vi "MccHat_extract_pressure_SPT25.vi"(8 "readings":cluster{i32, i32, dbl}[](array[cluster]), 11 "time":timestamp) -> (2 "P":dbl, 3 "waveform_array":waveform(dbl)[](array[waveform])=[{"t0"=timestamp(0 s since 1904-01-01), "dt"=1.0, "Y"=[]}, {"t0"=timestamp(3732035173.078092 s since 1904-01-01), "dt"=1.0, "Y"=[302.8589782714844], "attributes"=variant("NI_ChannelName"=variant(string "T1"))}])   [LabVIEW 2019]
panel:
  in  "V_max":dbl=10.0
  in  "V_min":dbl
  in  "P_max":dbl=30.0
  in  "P_min":dbl=-14.7
  out "V":dbl
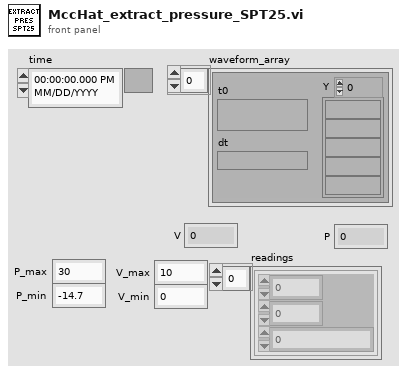
[diagram p1: front panel]
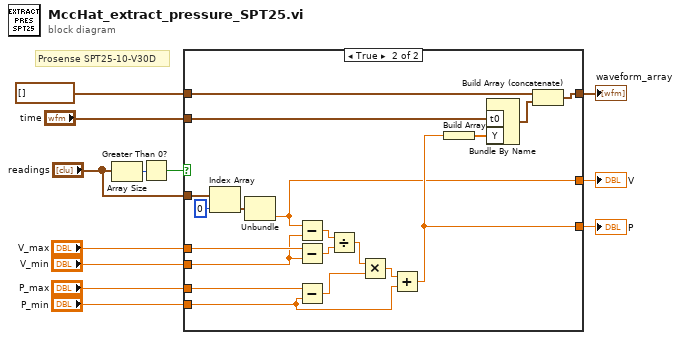
[diagram p0: block diagram]
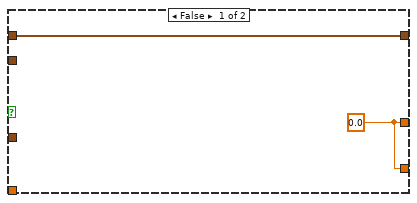
[diagram p2: hidden frame]
diagram:
  # "Prosense SPT25-10-V30D"
  n1 = Array Size(array="readings") -> (size(s)=w2:i32)
  n2 = Greater Than 0?(x=w2) -> (x > 0?=w12:bool)
  n3 = case shown="True" w12 {
    tunnel: waveform(dbl)[] [] -> [w14 w33]
    tunnel: "time" -> [_ w32]
    tunnel: [w14 w31] -> w9
    tunnel: [w13 w19] -> w8
    tunnel: [w13 w15] -> w7
    tunnel: "P_min" -> [_ w20]
    tunnel: "P_max" -> [_ w24]
    tunnel: "V_max" -> [_ w28]
    tunnel: "V_min" -> [_ w27]
    tunnel: "readings" -> [_ w18]
    frame False {
      w13 = 0.0 ("CJC (K)")
    }
    frame True {
      n4 = Index Array(array=w18, index=0) -> (element=w16:cluster{i32, i32, dbl})
      n5 = Unbundle(w16) -> (w15:dbl)  [unwired: 2 out]
      n6 = Subtract(x=w15, y=w27) -> (x-y=w25:dbl)
      n7 = Subtract(x=w28, y=w27) -> (x-y=w26:dbl)
      n8 = Subtract(x=w24, y=w20) -> (x-y=w23:dbl)
      n9 = Divide(x=w25, y=w26) -> (x/y=w22:dbl)
      n10 = Multiply(x=w22, y=w23) -> (x*y=w21:dbl)
      n11 = Add(x=w21, y=w20) -> (x+y=w19:dbl)
      n12 = Build Array(w19) -> (w30:dbl[])
      n13 = Bundle By Name("t0"=w32, "Y"=w30) -> (w29:waveform(dbl))  [unwired: 1 in]
      n14 = Build Array (concatenate)(w33, w29) -> (w31:waveform(dbl)[])
    }
  }
  "waveform_array" <- w9
  "P" <- w8
  "V" <- w7
